vi "Variant To Array Of Variants.vi"(6 "Variant":variant, 8 "error in (no error)":errorcluster, 11 "Registry Variant Accessor in":refnum<class "CConfig Variant Accessor.lvclass">) -> (0 "error out":errorcluster, 1 "Type Enum [auto]":T1, 3 "Registry Variant Accessor out":refnum<class "CConfig Variant Accessor.lvclass">, 4 "Variants":variant[](array[variant]), 5 "Types":T1[](array[typedef]), 7 "Labels (RAW)":string[](array[string]))   [LabVIEW 2013, in "CConfig Variant Accessor.lvclass"]
doc: "Copyright 2018, Carya Automatisering, Wiebe Walstra."
uses:
  CConfig Variant Accessor.lvclass
  <vilib>/Utility/VariantDataType/Type.ctl
  <vilib>/Utility/VariantDataType/VariantType.lvlib
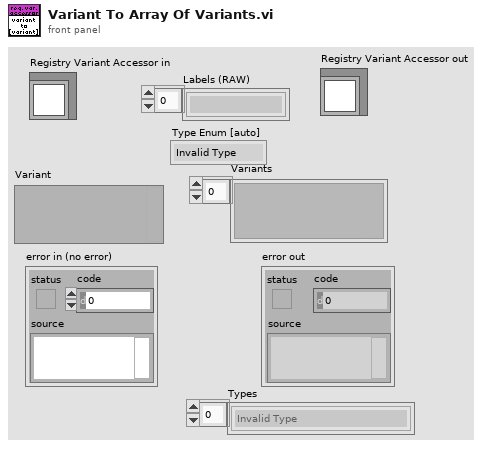
[diagram p1: front panel]
types:
  T1 = typedef "VariantType.lvlib/Type.ctl" = enum8{"Invalid Type", "Void", "I8", "I16", "I32", "I64", "U8", "U16", "U32", "U64", "Single Float", "Double Float", "Extended Float", "Single Complex", "Double Complex", "Extended Complex", "Enum U8", "Enum U16", "Enum U32", "Enum U64", "Single Float With Unit", "Double Float With Unit", "Extended Float With Unit", "Single Complex with Unit", "Double Complex with Unit", "Extended Complex with Unit", "Boolean", "String", "Path", "Picture", "Tag", "Array", "Cluster", "Variant", "LV Variant", "Waveform", "Timestamp", "Digital Waveform", "Digital Data", "ExpressData", "Refnum", "External Data", "VI", "Poly VI", "LabVIEW Class Instance", "Fixed Point"}
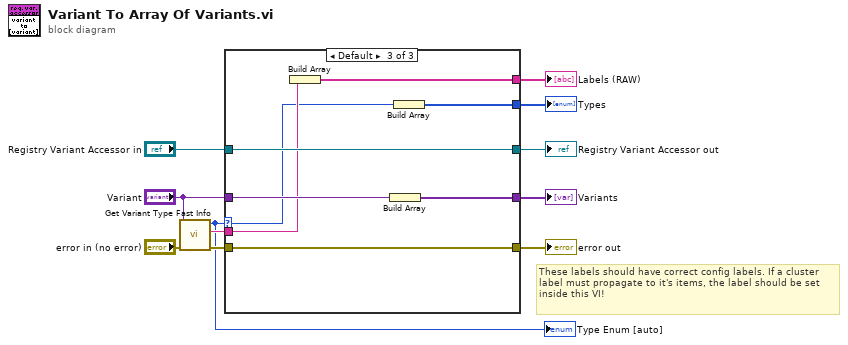
[diagram p0: block diagram]
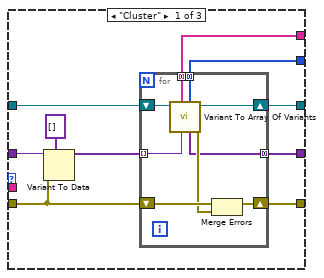
[diagram p2: hidden frame]
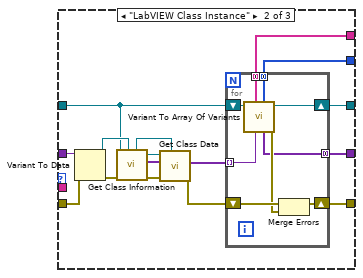
[diagram p3: hidden frame]
diagram:
  # "These labels should have correct config labels. If a cluster label must propagate to it's items, the label should be set inside this VI!"
  n1 = call "Get Variant Type Fast Info.vi"("error in (no error)"="error in (no error)", "Variant"="Variant") -> ("error out"=w11:errorcluster, "Name"=w2:string, "Type Enum"=w1:T1)  [unwired: 5 in, 2 out]
  "Type Enum [auto]" <- w1
  n2 = case shown="Default" w1 {
    selector: w1 -> [_ _ w57]
    tunnel: [w16 w45 w60] -> w8
    tunnel: w11 -> [w14 w32 w60]
    tunnel: "Registry Variant Accessor in" -> [w21 w38 w61]
    tunnel: [w20 w46 w61] -> w9
    tunnel: "Variant" -> [w17 w41 w63]
    tunnel: [w15 w44 w62] -> w5
    tunnel: w2 -> [_ _ w59]
    tunnel: [w13 w43 w58] -> w4
    tunnel: [w12 w42 w56] -> w3
    frame "Cluster" {
      n3 = Variant To Data(error in=w14, type=variant[] [], Variant=w17) -> (data=w18:variant[])  [unwired: 1 out]
      n4 = for {
        tunnel: w18 -> [w25] mode=indexing
        shift-right: [w27] -> w16
        shift-left: w14 -> [w28]
        shift-right: [w29] -> w20
        shift-left: w21 -> [w30]
        tunnel: [w22] -> w15 mode=concatenating
        tunnel: [w23] -> w13 mode=concatenating
        tunnel: [w24] -> w12 mode=concatenating
        n5 = call-dynamic "Variant To Array Of Variants.vi"("Variant"=w25, "Registry Variant Accessor in"=w30) -> ("error out"=w26:errorcluster, "Registry Variant Accessor out"=w29:refnum<class "CConfig Variant Accessor.lvclass">, "Variants"=w22:variant[], "Types"=w24:T1[], "Labels (RAW)"=w23:string[])  [unwired: 4 in, 1 out]
        n6 = Merge Errors(w28, w26) -> (w27:errorcluster)
      }
    }
    frame "LabVIEW Class Instance" {
      n7 = Variant To Data(error in=w32, Variant=w41) -> (data=w39:refnum<class>, error out=w37:errorcluster)  [unwired: 1 in]
      n8 = call "Get Class Information.vi"("Object"=w39, "error in (no error)"=w37, "CConfig Variant Accessor in"=w38) -> ("error out"=w35:errorcluster, "Class default data"=w36:variant[], "CConfig Variant Accessor out"=w34:refnum<class "CConfig Variant Accessor.lvclass">, "Object (dup)"=w33:refnum<class>)  [unwired: 3 in, 2 out]
      n9 = call "Get Class Data.vi"("Object"=w33, "error in (no error)"=w35, "Class default data"=w36, "CConfig Variant Accessor in"=w34) -> ("error out"=w31:errorcluster, "Class data"=w40:variant[])  [unwired: 4 in, 2 out]
      n10 = for {
        shift-right: [w52] -> w45
        shift-left: w31 -> [w53]
        shift-right: [w54] -> w46
        shift-left: w38 -> [w55]
        tunnel: [w48] -> w44 mode=concatenating
        tunnel: [w49] -> w43 mode=concatenating
        tunnel: [w50] -> w42 mode=concatenating
        tunnel: w40 -> [w47] mode=indexing
        n11 = call-dynamic "Variant To Array Of Variants.vi"("Variant"=w47, "Registry Variant Accessor in"=w55) -> ("error out"=w51:errorcluster, "Registry Variant Accessor out"=w54:refnum<class "CConfig Variant Accessor.lvclass">, "Variants"=w48:variant[], "Types"=w50:T1[], "Labels (RAW)"=w49:string[])  [unwired: 4 in, 1 out]
        n12 = Merge Errors(w53, w51) -> (w52:errorcluster)
      }
    }
    frame Default {
      n13 = Build Array(w59) -> (w58:string[])
      n14 = Build Array(w63) -> (w62:variant[])
      n15 = Build Array(w57) -> (w56:T1[])
    }
  }
  "error out" <- w8
  "Registry Variant Accessor out" <- w9
  "Variants" <- w5
  "Labels (RAW)" <- w4
  "Types" <- w3
